vi "parse gentec acquire string.vi"(11 "Acquisition String":string) -> (2 "Channel 2 value":dbl, 3 "Channel 1 value":dbl)   [LabVIEW 2020, in "Gentec SlinkUSB.lvclass"]
uses:
  Gentec SlinkUSB.lvclass
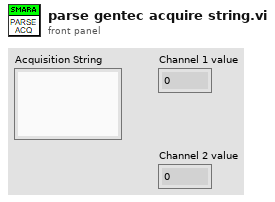
[diagram p1: front panel]
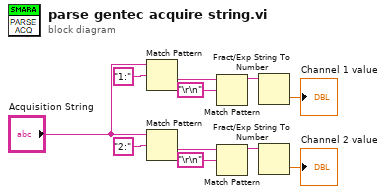
[diagram p0: block diagram]
diagram:
  n1 = Match Pattern(string="Acquisition String", regular expression="1:") -> (after substring=w5:string)  [unwired: 1 in, 3 out]
  n2 = Match Pattern(string="Acquisition String", regular expression="2:") -> (after substring=w10:string)  [unwired: 1 in, 3 out]
  n3 = Match Pattern(string=w5, regular expression="\r\n") -> (before substring=w6:string)  [unwired: 1 in, 3 out]
  n4 = Match Pattern(string=w10, regular expression="\r\n") -> (before substring=w11:string)  [unwired: 1 in, 3 out]
  n5 = Fract/Exp String To Number(string=w6) -> (number=→"Channel 1 value":dbl)  [unwired: 3 in, 1 out]
  n6 = Fract/Exp String To Number(string=w11) -> (number=→"Channel 2 value":dbl)  [unwired: 3 in, 1 out]
